vi "截取字符串（二进）.vi"(3 "长度":i32[](array[numeric]), 4 "数组 2":i32[](array[numeric]), 5 "数组1":i32[](array[numeric])) -> (1 "子数组2":i32[](array[numeric]), 2 "子数组1":i32[](array[numeric]))   [LabVIEW 2019]
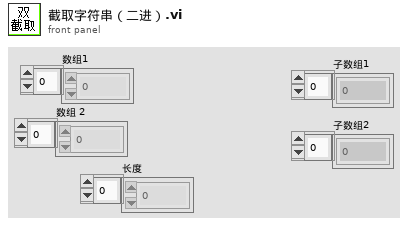
[diagram p1: front panel]
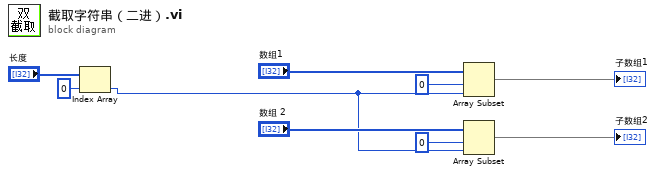
[diagram p0: block diagram]
diagram:
  n1 = Index Array(array="长度", index=0 ("索引")) -> (element=w1:i32)
  n2 = Array Subset(array="数组1", index=0 ("索引"), length=w1) -> (→"子数组1":i32[])
  n3 = Array Subset(array="数组 2", index=0 ("索引"), length=w1) -> (→"子数组2":i32[])
